vi "fgv_ycar_opval.vi"(7 "cmd":enum16{"read", "write", "ini"}(ring), 11 "opval":cluster{"speed":dbl, "steer":dbl}) -> (3 "opval out":cluster{"speed":dbl, "steer":dbl})   [LabVIEW 2019]
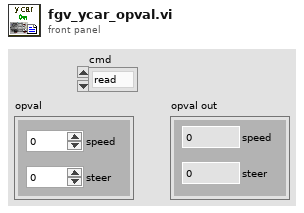
[diagram p1: front panel]
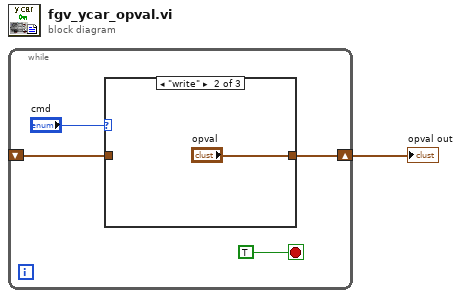
[diagram p0: block diagram]
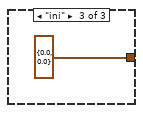
[diagram p3: hidden frame]
diagram:
  n1 = while {
    shift-right: [w3] -> w1
    shift-left: _ -> [w2]
    stop <- TRUE stop-if-true
    n2 = case shown="\"write\"" "cmd" {
      tunnel: [w6 "opval" cluster{"speed":dbl, "steer":dbl} {"speed"=0.0, "steer"=0.0} ("opval")] -> w3
      tunnel: w2 -> [w6 _ _]
      frame "read", Default {
      }
      frame "write" {
      }
      frame "ini" {
      }
    }
  }
  "opval out" <- w1
